vi "Global.vi"() -> ()   [LabVIEW 2021]
panel:
  in  "System Net Current (A)":dbl
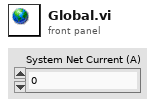
[diagram p1: front panel]
diagram:
